vi "get model data interface.vi"(8 "error in":errorcluster, 11 "new VI path":path) -> (0 "error out":errorcluster, 1 "parameters":T1[](array[typedef]), 2 "indicators":T1[](array[typedef]), 3 "controls":T1[](array[typedef]), 5 "vi reference":refnum<vi>)   [LabVIEW 2014, in "CD model script.lvlib"]
uses:
  CD model script.lvlib
  interface spec.ctl
  <vilib>/Utility/VariantDataType/VariantType.lvlib
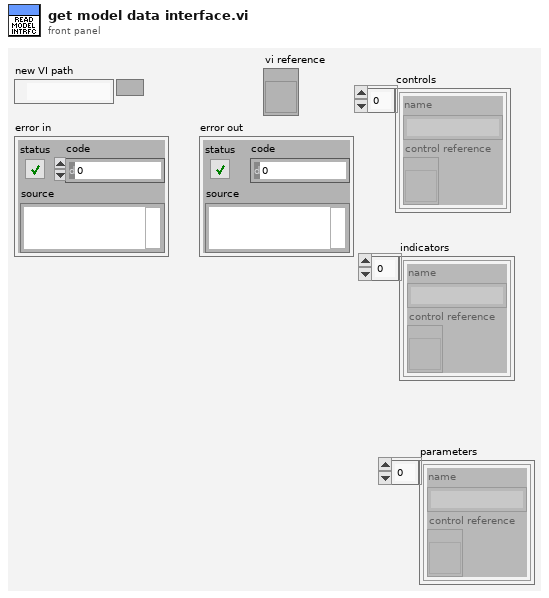
[diagram p1: front panel]
types:
  T1 = typedef "CD model script.lvlib/interface spec.ctl" = cluster{"name":string, "control reference":refnum<vi>}
  T2 = typedef "VariantType.lvlib/Type.ctl" = enum8{"Invalid Type", "Void", "I8", "I16", "I32", "I64", "U8", "U16", "U32", "U64", "Single Float", "Double Float", "Extended Float", "Single Complex", "Double Complex", "Extended Complex", "Enum U8", "Enum U16", "Enum U32", "Enum U64", "Single Float With Unit", "Double Float With Unit", "Extended Float With Unit", "Single Complex with Unit", "Double Complex with Unit", "Extended Complex with Unit", "Boolean", "String", "Path", "Picture", "Tag", "Array", "Cluster", "Variant", "LV Variant", "Waveform", "Timestamp", "Digital Waveform", "Digital Data", "ExpressData", "Refnum", "External Data", "VI", "Poly VI", "LabVIEW Class Instance", "Fixed Point"}
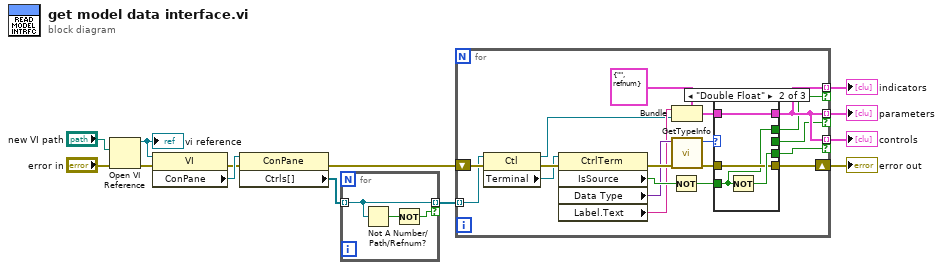
[diagram p0: block diagram]
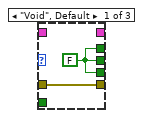
[diagram p2: hidden frame]
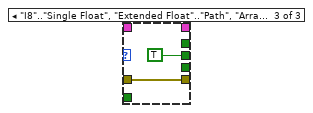
[diagram p3: hidden frame]
diagram:
  n1 = Open VI Reference(vi path="new VI path", error in (no error)="error in") -> (vi reference=w10:refnum<vi>, error out=w11:errorcluster)  [unwired: 4 in]
  "vi reference" <- w10
  n2 = property class="VI"(reference=w10, error in=w11) -> (error out=w8:errorcluster, "ConPane"=w9:refnum<vi>)  [unwired: 1 out]
  n3 = property class="ConPane"(reference=w9, error in=w8) -> (error out=w7:errorcluster, "Ctrls[]"=w2:refnum<vi>[])  [unwired: 1 out]
  n4 = for {
    tunnel: w2 -> [w15] mode=indexing
    tunnel: [w15] -> w1 mode=indexing if=w14
    n5 = Not A Number/Path/Refnum?(number/path/refnum=w15) -> (NaN/Path/Refnum?=w16:bool)
    n6 = Not(x=w16) -> (.not. x?=w14:bool)
  }
  n7 = for {
    shift-right: [w31] -> w6
    shift-left: w7 -> [w35]
    tunnel: w1 -> [w20] mode=indexing
    tunnel: [w29] -> w5 mode=indexing if=w27
    tunnel: [w29] -> w4 mode=indexing if=w28
    tunnel: [w29] -> w3 mode=indexing if=w22
    n8 = property class="Ctl"(reference=w20, error in=w35) -> (reference out=w17:refnum<vi>, error out=w21:errorcluster, "Terminal"=w19:refnum<vi>)
    n9 = property class="CtrlTerm"(reference=w19, error in=w21) -> (error out=w34:errorcluster, "IsSource"=w30:bool, "Data Type"=w26:variant, "Label.Text"=w24:string)  [unwired: 1 out]
    n10 = Not(x=w30) -> (.not. x?=w18:bool)
    n11 = Bundle(cluster=T1 {"name"="", "control reference"=refnum} ("interface spec"), "name"=w24, "control reference"=w17) -> (w23:T1)
    n12 = call <vilib>:"GetTypeInfo.vi"("error in (no error)"=w34, "Variant"=w26) -> ("error out"=w32:errorcluster, "Type Enum"=w33:T2)  [unwired: 5 in, 3 out]
    n13 = case shown="\"Double Float\"" w33 {
      tunnel: w32 -> [w36 w40 w43]
      tunnel: [w37 w41 _] -> w27
      tunnel: [w37 w39 _] -> w28
      tunnel: [w37 _ TRUE] -> w22
      tunnel: [w36 w40 w43] -> w31
      tunnel: w18 -> [_ w39 _]
      tunnel: [_ w38 _] -> w29
      tunnel: w23 -> [_ w38 _]
      frame "Void", Default {
        w37 = FALSE
      }
      frame "Double Float" {
        n14 = Not(x=w39) -> (.not. x?=w41:bool)
      }
      frame "I8".."Single Float", "Extended Float".."Path", "Array", "Cluster" {
      }
    }
  }
  "error out" <- w6
  "controls" <- w5
  "indicators" <- w4
  "parameters" <- w3
